vi "SingleStructRead.vi"() -> ()   [LabVIEW 2022 SP3]
uses:
  <userlib>/Beckhoff-LabVIEW-Interface/_DependsOn/Base/Read/Read Sync.vi
  <userlib>/Beckhoff-LabVIEW-Interface/_DependsOn/Base/TypeResolver/Get TypeResolver.vi
panel:
  out "error out":errorcluster
  in  "error in":errorcluster
  out "RDataArray":variant[](array[variant])
  out "Read status?":bool
  in  "String":string
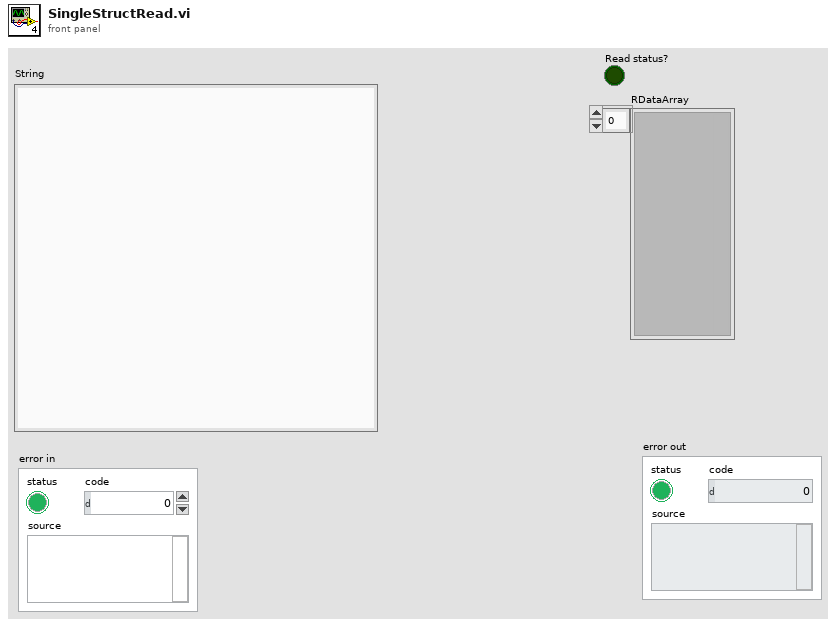
[diagram p1: front panel]
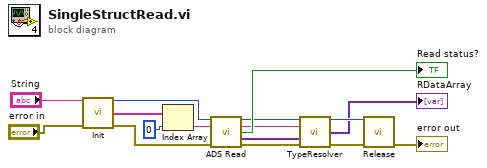
[diagram p0: block diagram]
diagram:
  n1 = call <userlib>:"Init.vi"("XMLDescription"="String", "error in (no error)"="error in") -> ("Handle"=w14:u32, "ReadGrpSymbols"=w13:string[], "error out"=w15:errorcluster)  [unwired: 9 in, 2 out]
  n2 = Index Array(array=w13, index=0) -> (element=w11:string)
  n3 = call-poly <userlib>:"ADS Read.vi"("Handle"=w14, "SymbolName"=w11, "error in (no error)"=w15) -> ("Handle"=w9:u32, "SymbolName"=w8:string, "Read status?"=→"Read status?":bool, "Ads Read Data"=w7:variant[], "error out"=w6:errorcluster)  [unwired: 8 in]
  n4 = call-poly <userlib>:"TypeResolver.vi"("Handle"=w9, "SymbolName"=w8, "ADSRData"=w7, "error in"=w6) -> ("Handle"=w4:u32, "RDataArray"=→"RDataArray":variant[], "error out"=w5:errorcluster)  [unwired: 8 in, 1 out]
  n5 = call <userlib>:"Release.vi"("Handle"=w4, "error in (no error)"=w5) -> ("error out"=→"error out":errorcluster)  [unwired: 13 in]
